vi "podControl_9066.vi"() -> ()   [LabVIEW 2015]
uses:
  <vilib>/platform/TimedLoop/XDataNode/XDataNode.xnode
  <vilib>/Platform/TimedLoop/XDataNode/nitl_modes.ctl
  <vilib>/Platform/TimedLoop/XDataNode/XDNodeRunTimeDep.lvlib
  <vilib>/Platform/TimedLoop/XDataNode/wakeup.ctl
  <vilib>/Platform/TimedLoop/XDataNode/timing_clust.ctl
  podGlobals_9066.vi
  <vilib>/Platform/TimedLoop/XDataNode/loadnilvce.vi
panel:
  out "L:":dbl
  out "Internal Pressure (atm)":dbl(slide) scale=0.0..2.0
  out "Internal Temperature (F)":dbl(slide) scale=50.0..120.0
  out "READY":bool
  out "Runtime (s)":dbl
  in  "START":bool
  out "R:":dbl
  out "Acceleration (m/s^2)":dbl(knob) scale=-30.0..30.0
  out "Position (m)":dbl
  out "Velocity (m/s)":dbl(knob) scale=0.0..300.0
  in  "Custom Profile Velocity (m/s)":dbl
  out "Door Open":bool
  out "Pusher Engaged":bool
  out "Front Brake Engaged":bool
  out "Back Brake Engaged":bool
  in  "Flight Profile":T1(radio)
  out "Progress":u8(slide) caption="Profile Progress" scale=0.0..100.0
  out "Battery Pressure (atm)":dbl(slide) scale=0.0..2.0
  out "Battery Temperature (F)":dbl(slide) scale=50.0..120.0
  in  "STOP":bool
  out "Battery 2 Voltage":dbl(knob) scale=22.0..26.0
  out "Battery 1 Voltage":dbl(knob) scale=22.0..26.0
  # "Z-Height (mm)"
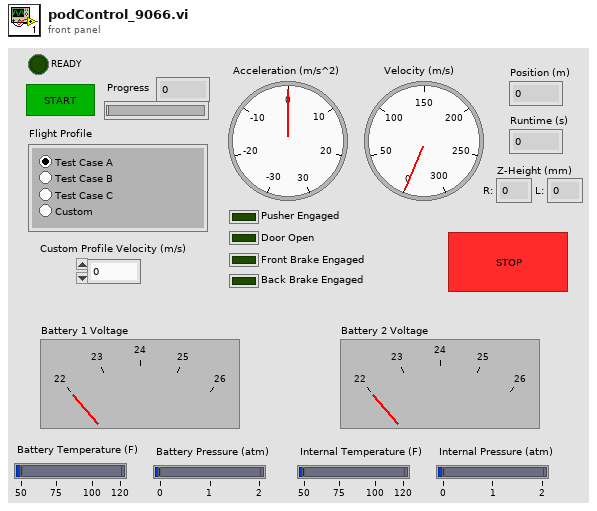
[diagram p1: front panel]
types:
  T1 = enum32{"20 MPH (Test Case A)", "60 MPH (Test Case B)", "150 MPH (Test Case C)", "Custom"}
  T2 = typedef "XDNodeRunTimeDep.lvlib/timing_clust.ctl" = cluster{"Expected End [f-1]":u64, "Actual End [f-1]":u64, "Finished Late? [f-1]":bool, "Expected End [i-1]":u64, "Actual End [i-1]":u64, "Finished Late? [i-1]":bool, "Expected Start [i]":u64, "Actual Start [i]":u64, "Expected Start [f]":u64, "Actual Start [f]":u64, "Source Name":string, "Structure Name":string, "Period":i64, "Deadline":i64, "Offset":i64, "Start":i64, "Priority":i32, "Timeout":i32, "Mode":T3, "Wakeup Reason":T4, "Error":errorcluster, "Source Type":string, "Secondary Source Type":string, "Global End Time":u64, "Global Start Time":u64, "Frame Duration":u64, "Iteration Duration":u64, "Assigned CPU":i32, "I/O Scan Engine Mode":u32}
  T3 = typedef "XDNodeRunTimeDep.lvlib/nitl_modes.ctl" = enum32{"No Change", "Process missed periods, maintain original phase", "Discard missed periods, maintain original phase", "Process missed periods, ignore original phase", "Discard missed periods, ignore original phase"}
  T4 = typedef "XDNodeRunTimeDep.lvlib/wakeup.ctl" = enum32{"Normal", "Aborted", "Asynchronous wakeup", "Timing source error", "Timed loop error", "Timeout"}
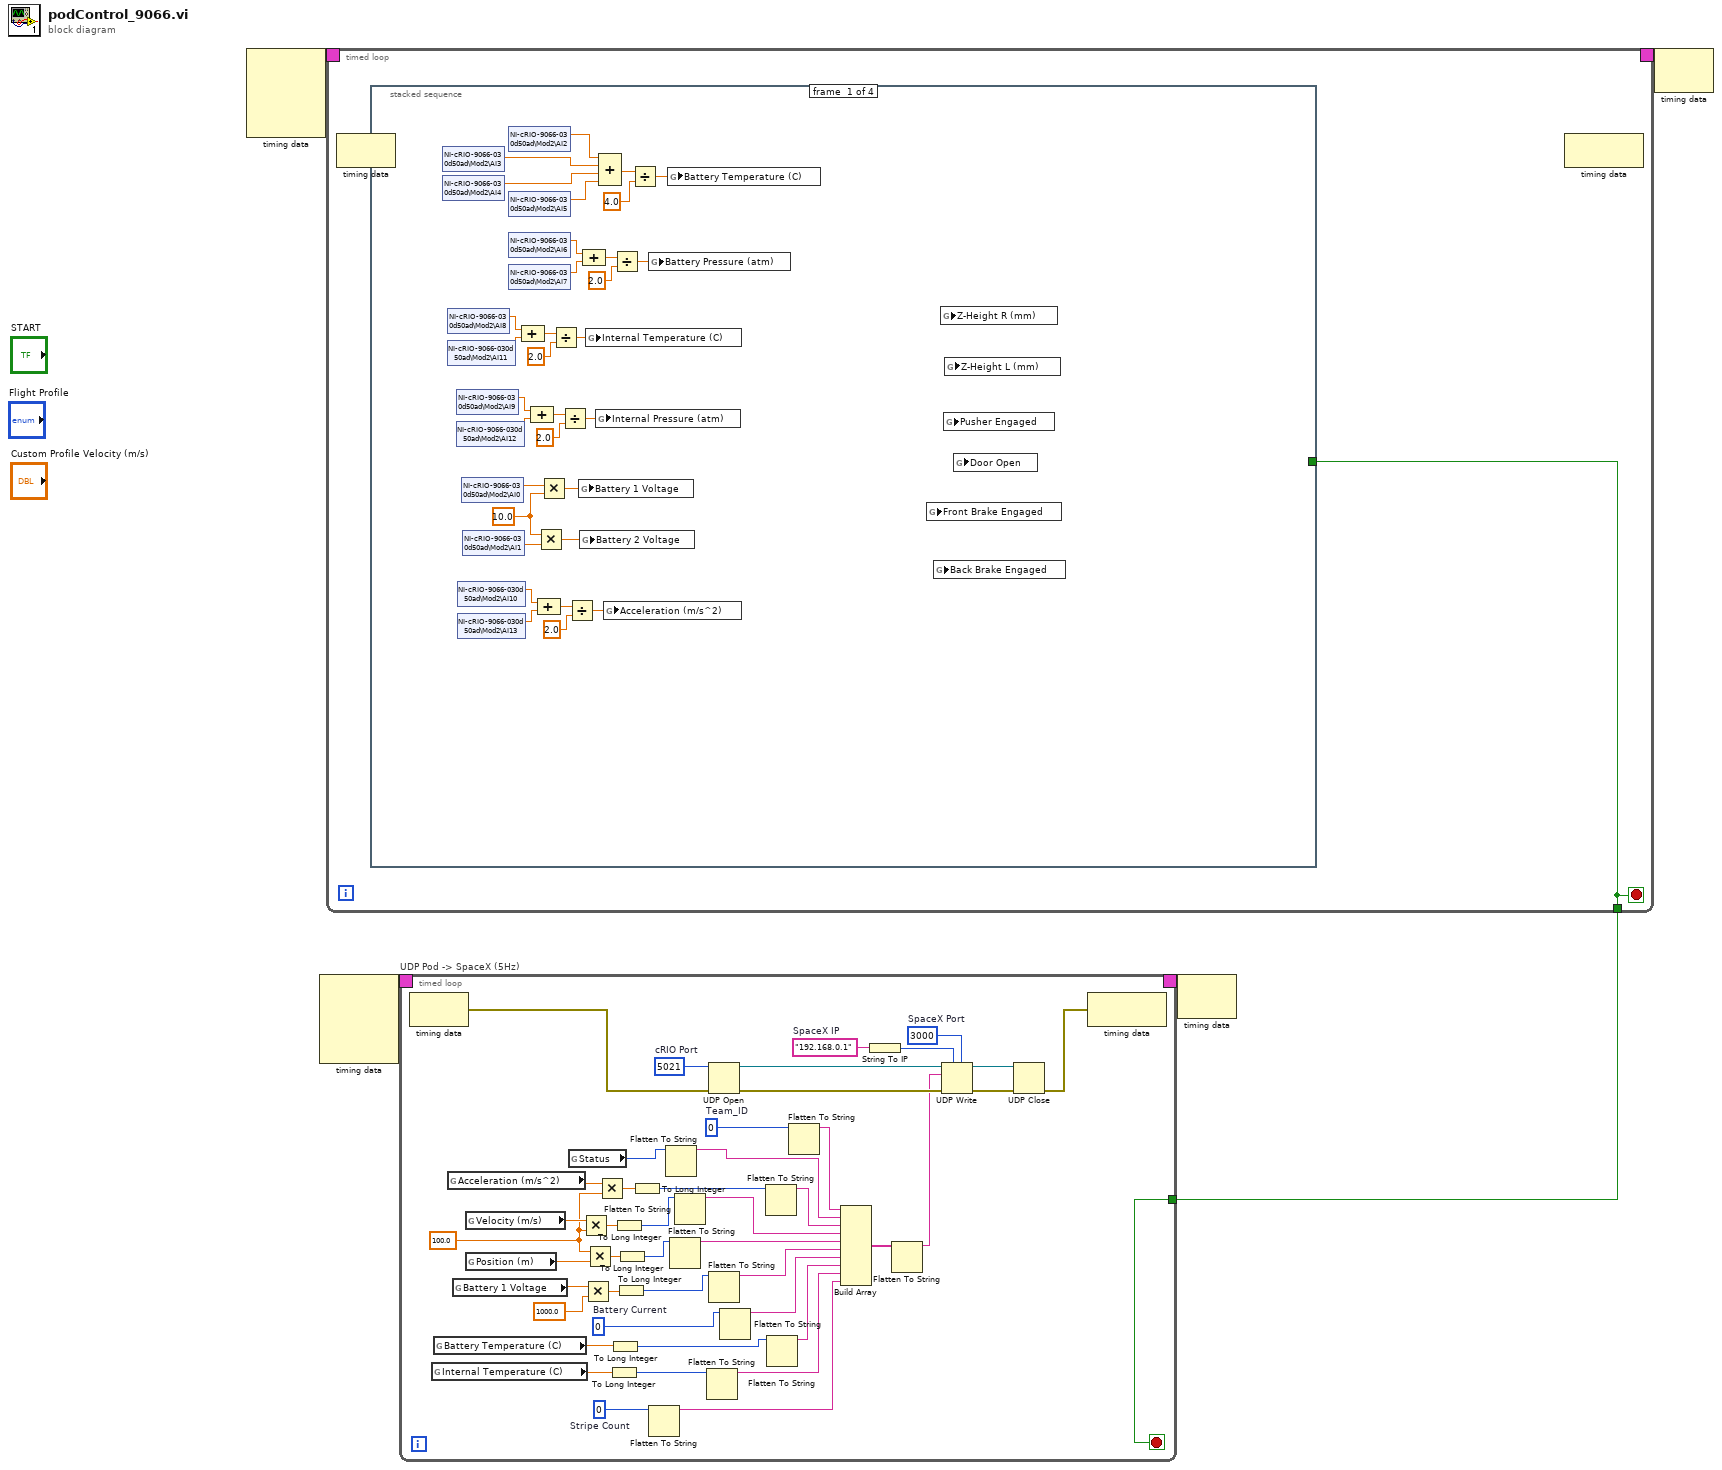
[diagram p0: block diagram]
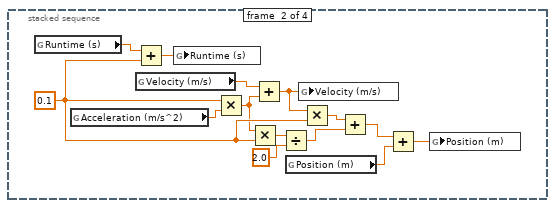
[diagram p2: hidden frame]
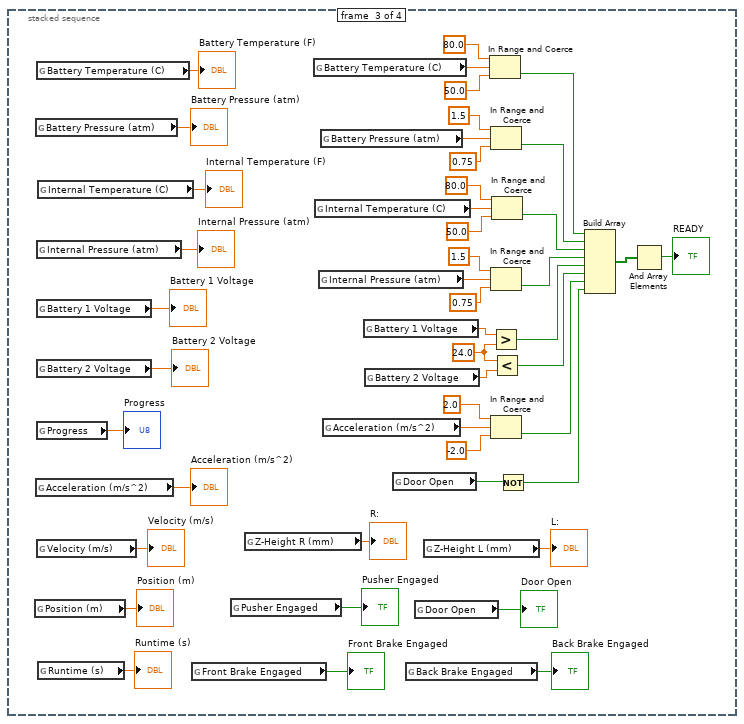
[diagram p3: hidden frame]
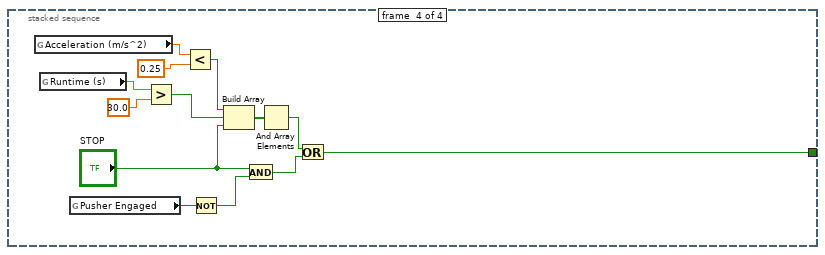
[diagram p4: hidden frame]
diagram:
  n1 = node-c288() -> (w5:T2)  [unwired: 4 in]
  n2 = node-c288() -> (w3:T2)  [unwired: 4 in]
  n3 = timed-loop {
    timing: w5 -> [_]
    timing-out: [_] -> w4
    tunnel: [w6] -> w1
    stop <- w6 stop-if-true
    n4 = node-c288() -> ()  [unwired: 1 in, 1 out]
    n5 = stacked-sequence {
      tunnel: [_ _ _ w106] -> w6
      frame #0 {
        w36 = 10.0
        n6 = shared-variable "NI-cRIO-9066-030d50ad\\Mod2\\AI3"() -> (w19:dbl)  [unwired: 1 in, 1 out]
        n7 = shared-variable "NI-cRIO-9066-030d50ad\\Mod2\\AI4"() -> (w20:dbl)  [unwired: 1 in, 1 out]
        n8 = shared-variable "NI-cRIO-9066-030d50ad\\Mod2\\AI8"() -> (w8:dbl)  [unwired: 1 in, 1 out]
        n9 = shared-variable "NI-cRIO-9066-030d50ad\\Mod2\\AI11"() -> (w9:dbl)  [unwired: 1 in, 1 out]
        n10 = shared-variable "NI-cRIO-9066-030d50ad\\Mod2\\AI9"() -> (w13:dbl)  [unwired: 1 in, 1 out]
        n11 = shared-variable "NI-cRIO-9066-030d50ad\\Mod2\\AI12"() -> (w14:dbl)  [unwired: 1 in, 1 out]
        n12 = shared-variable "NI-cRIO-9066-030d50ad\\Mod2\\AI10"() -> (w29:dbl)  [unwired: 1 in, 1 out]
        n13 = shared-variable "NI-cRIO-9066-030d50ad\\Mod2\\AI13"() -> (w30:dbl)  [unwired: 1 in, 1 out]
        n14 = shared-variable "NI-cRIO-9066-030d50ad\\Mod2\\AI0"() -> (w34:dbl)  [unwired: 1 in, 1 out]
        n15 = shared-variable "NI-cRIO-9066-030d50ad\\Mod2\\AI1"() -> (w35:dbl)  [unwired: 1 in, 1 out]
        n16 = shared-variable "NI-cRIO-9066-030d50ad\\Mod2\\AI2"() -> (w7:dbl)  [unwired: 1 in, 1 out]
        n17 = shared-variable "NI-cRIO-9066-030d50ad\\Mod2\\AI5"() -> (w21:dbl)  [unwired: 1 in, 1 out]
        n18 = shared-variable "NI-cRIO-9066-030d50ad\\Mod2\\AI6"() -> (w24:dbl)  [unwired: 1 in, 1 out]
        n19 = shared-variable "NI-cRIO-9066-030d50ad\\Mod2\\AI7"() -> (w25:dbl)  [unwired: 1 in, 1 out]
        n20 = Compound Arithmetic op=ADD(w8, w9) -> (w10:dbl)
        n21 = Compound Arithmetic op=ADD(w13, w14) -> (w15:dbl)
        n22 = Multiply(x=w36, y=w35) -> (x*y=w38:dbl)
        n23 = Compound Arithmetic op=ADD(w29, w30) -> (w31:dbl)
        n24 = Multiply(x=w34, y=w36) -> (x*y=w37:dbl)
        n25 = Divide(x=w10, y=2.0) -> (x/y=w12:dbl)
        n26 = Divide(x=w15, y=2.0) -> (x/y=w17:dbl)
        n27 = Divide(x=w31, y=2.0) -> (x/y=w33:dbl)
        n28 = global write "podGlobals_9066.vi" "Battery 1 Voltage"(w37) -> ()
        n29 = global write "podGlobals_9066.vi" "Battery 2 Voltage"(w38) -> ()
        n30 = Compound Arithmetic op=ADD(w24, w25) -> (w26:dbl)
        n31 = global write "podGlobals_9066.vi" "Internal Temperature (C)"(w12) -> ()
        n32 = global write "podGlobals_9066.vi" "Internal Pressure (atm)"(w17) -> ()
        n33 = Compound Arithmetic op=ADD(w7, w19, w20, w21) -> (w18:dbl)
        n34 = global write "podGlobals_9066.vi" "Acceleration (m/s^2)"(w33) -> ()
        n35 = Divide(x=w26, y=2.0) -> (x/y=w28:dbl)
        n36 = Divide(x=w18, y=4.0) -> (x/y=w23:dbl)
        n37 = global write "podGlobals_9066.vi" "Battery Pressure (atm)"(w28) -> ()
        n38 = global write "podGlobals_9066.vi" "Battery Temperature (C)"(w23) -> ()
        n39 = global read "podGlobals_9066.vi" "Front Brake Engaged"() -> ()  [unwired: 1 in]
        n40 = global read "podGlobals_9066.vi" "Back Brake Engaged"() -> ()  [unwired: 1 in]
        n41 = global read "podGlobals_9066.vi" "Z-Height R (mm)"() -> ()  [unwired: 1 in]
        n42 = global read "podGlobals_9066.vi" "Pusher Engaged"() -> ()  [unwired: 1 in]
        n43 = global read "podGlobals_9066.vi" "Z-Height L (mm)"() -> ()  [unwired: 1 in]
        n44 = global read "podGlobals_9066.vi" "Door Open"() -> ()  [unwired: 1 in]
      }
      frame #1 {
        w51 = 0.1
        n45 = global read "podGlobals_9066.vi" "Runtime (s)"() -> (w40:dbl)
        n46 = global read "podGlobals_9066.vi" "Acceleration (m/s^2)"() -> (w49:dbl)
        n47 = Add(x=w40, y=w51) -> (x+y=w39:dbl)
        n48 = global read "podGlobals_9066.vi" "Velocity (m/s)"() -> (w41:dbl)
        n49 = global write "podGlobals_9066.vi" "Runtime (s)"(w39) -> ()
        n50 = Multiply(x=w51, y=w49) -> (x*y=w43:dbl)
        n51 = Multiply(x=w43, y=w51) -> (x*y=w44:dbl)
        n52 = Add(x=w41, y=w43) -> (x+y=w52:dbl)
        n53 = Divide(x=w44, y=2.0) -> (x/y=w47:dbl)
        n54 = global read "podGlobals_9066.vi" "Position (m)"() -> (w46:dbl)
        n55 = global write "podGlobals_9066.vi" "Velocity (m/s)"(w52) -> ()
        n56 = Multiply(x=w52, y=w51) -> (x*y=w50:dbl)
        n57 = Add(x=w50, y=w47) -> (x+y=w48:dbl)
        n58 = Add(x=w48, y=w46) -> (x+y=w42:dbl)
        n59 = global write "podGlobals_9066.vi" "Position (m)"(w42) -> ()
      }
      frame #2 {
        w72 = 24.0
        n60 = global read "podGlobals_9066.vi" "Position (m)"() -> (→"Position (m)":dbl)
        n61 = global read "podGlobals_9066.vi" "Battery Pressure (atm)"() -> (→"Battery Pressure (atm)":dbl)
        n62 = global read "podGlobals_9066.vi" "Acceleration (m/s^2)"() -> (→"Acceleration (m/s^2)":dbl)
        n63 = global read "podGlobals_9066.vi" "Battery Temperature (C)"() -> (→"Battery Temperature (F)":dbl)
        n64 = global read "podGlobals_9066.vi" "Internal Pressure (atm)"() -> (→"Internal Pressure (atm)":dbl)
        n65 = global read "podGlobals_9066.vi" "Battery 1 Voltage"() -> (→"Battery 1 Voltage":dbl)
        n66 = global read "podGlobals_9066.vi" "Battery 2 Voltage"() -> (→"Battery 2 Voltage":dbl)
        n67 = global read "podGlobals_9066.vi" "Progress"() -> (→"Progress":dbl)
        n68 = global read "podGlobals_9066.vi" "Velocity (m/s)"() -> (→"Velocity (m/s)":dbl)
        n69 = global read "podGlobals_9066.vi" "Internal Temperature (C)"() -> (→"Internal Temperature (F)":dbl)
        n70 = global read "podGlobals_9066.vi" "Runtime (s)"() -> (→"Runtime (s)":dbl)
        n71 = global read "podGlobals_9066.vi" "Front Brake Engaged"() -> (→"Front Brake Engaged":bool)
        n72 = global read "podGlobals_9066.vi" "Pusher Engaged"() -> (→"Pusher Engaged":bool)
        n73 = global read "podGlobals_9066.vi" "Z-Height R (mm)"() -> (→"R:":dbl)
        n74 = global read "podGlobals_9066.vi" "Battery Temperature (C)"() -> (w61:dbl)
        n75 = global read "podGlobals_9066.vi" "Internal Temperature (C)"() -> (w55:dbl)
        n76 = global read "podGlobals_9066.vi" "Internal Pressure (atm)"() -> (w58:dbl)
        n77 = global read "podGlobals_9066.vi" "Battery Pressure (atm)"() -> (w64:dbl)
        n78 = global read "podGlobals_9066.vi" "Acceleration (m/s^2)"() -> (w67:dbl)
        n79 = global read "podGlobals_9066.vi" "Battery 1 Voltage"() -> (w70:dbl)
        n80 = global read "podGlobals_9066.vi" "Battery 2 Voltage"() -> (w71:dbl)
        n81 = global read "podGlobals_9066.vi" "Door Open"() -> (w80:bool)
        n82 = global read "podGlobals_9066.vi" "Back Brake Engaged"() -> (→"Back Brake Engaged":bool)
        n83 = global read "podGlobals_9066.vi" "Door Open"() -> (→"Door Open":bool)
        n84 = global read "podGlobals_9066.vi" "Z-Height L (mm)"() -> (→"L:":dbl)
        n85 = In Range and Coerce(upper limit=80.0, x=w61, lower limit=50.0) -> (In Range?=w73:bool)  [unwired: 1 out]
        n86 = In Range and Coerce(upper limit=1.5, x=w64, lower limit=0.75) -> (In Range?=w74:bool)  [unwired: 1 out]
        n87 = In Range and Coerce(upper limit=1.5, x=w58, lower limit=0.75) -> (In Range?=w76:bool)  [unwired: 1 out]
        n88 = Greater?(x=w70, y=w72) -> (0:w77:bool)
        n89 = In Range and Coerce(upper limit=2.0, x=w67, lower limit=-2.0) -> (In Range?=w79:bool)  [unwired: 1 out]
        n90 = In Range and Coerce(upper limit=80.0, x=w55, lower limit=50.0) -> (In Range?=w75:bool)  [unwired: 1 out]
        n91 = Less?(x=w72, y=w71) -> (x < y?=w78:bool)
        n92 = Not(x=w80) -> (.not. x?=w81:bool)
        n93 = Build Array(w73, w74, w75, w76, w77, w78, w79, w81) -> (w53:bool[])
        n94 = And Array Elements(Boolean array=w53) -> (logical AND=→"READY":bool)
      }
      frame #3 {
        n95 = global read "podGlobals_9066.vi" "Acceleration (m/s^2)"() -> (w103:dbl)
        n96 = global read "podGlobals_9066.vi" "Runtime (s)"() -> (w108:dbl)
        n97 = global read "podGlobals_9066.vi" "Pusher Engaged"() -> (w111:bool)
        n98 = Greater?(x=w108, y=30.0) -> (0:w101:bool)
        n99 = Less?(x=w103, y=0.25) -> (x < y?=w99:bool)
        n100 = Not(x=w111) -> (.not. x?=w110:bool)
        n101 = Build Array(w99, w101, "STOP") -> (w105:bool[])
        n102 = And(x="STOP", y=w110) -> (x .and. y?=w109:bool)
        n103 = And Array Elements(Boolean array=w105) -> (logical AND=w104:bool)
        n104 = Or(x=w104, y=w109) -> (x .or. y?=w106:bool)
      }
    }
    n105 = node-c288() -> ()  [unwired: 1 in, 1 out]
  }
  n106 = timed-loop "UDP Pod -> SpaceX (5Hz)" {
    timing: w3 -> [_]
    timing-out: [_] -> w2
    tunnel: w1 -> [w114]
    stop <- w114 stop-if-true
    w119 = u32 0  # Stripe Count
    w125 = 0  # Battery Current
    w146 = 100.0
    w137 = u8 0  # Team_ID
    w151 = 3000  # SpaceX Port
    w115 = "192.168.0.1"  # SpaceX IP
    w154 = 5021  # cRIO Port
    n107 = node-c288() -> (w158:errorcluster)  [unwired: 1 in]
    n108 = global read "podGlobals_9066.vi" "Internal Temperature (C)"() -> (w138:dbl)
    n109 = global read "podGlobals_9066.vi" "Battery Temperature (C)"() -> (w139:dbl)
    n110 = global read "podGlobals_9066.vi" "Acceleration (m/s^2)"() -> (w149:dbl)
    n111 = global read "podGlobals_9066.vi" "Battery 1 Voltage"() -> (w140:dbl)
    n112 = global read "podGlobals_9066.vi" "Velocity (m/s)"() -> (w148:dbl)
    n113 = global read "podGlobals_9066.vi" "Position (m)"() -> (w147:dbl)
    n114 = global read "podGlobals_9066.vi" "Status"() -> (w135:u8)
    n115 = Multiply(x=w148, y=w146) -> (x*y=w144:dbl)
    n116 = Multiply(x=w140, y=1000.0) -> (x*y=w142:dbl)
    n117 = Multiply(x=w146, y=w147) -> (x*y=w143:dbl)
    n118 = Multiply(x=w149, y=w146) -> (x*y=w145:dbl)
    n119 = To Long Integer(number=w138) -> (32bit integer=w121:i32)
    n120 = To Long Integer(number=w139) -> (32bit integer=w123:i32)
    n121 = To Long Integer(number=w144) -> (32bit integer=w130:i32)
    n122 = To Long Integer(number=w142) -> (32bit integer=w127:i32)
    n123 = To Long Integer(number=w143) -> (32bit integer=w128:i32)
    n124 = To Long Integer(number=w145) -> (32bit integer=w132:i32)
    n125 = Flatten To String(anything=w119) -> (data string=w118:string)  [unwired: 3 in, 2 out]
    n126 = Flatten To String(anything=w135) -> (data string=w134:string)  [unwired: 3 in, 2 out]
    n127 = Flatten To String(anything=w128) -> (data string=w129:string)  [unwired: 3 in, 2 out]
    n128 = Flatten To String(anything=w130) -> (data string=w131:string)  [unwired: 3 in, 2 out]
    n129 = Flatten To String(anything=w121) -> (data string=w120:string)  [unwired: 3 in, 2 out]
    n130 = UDP Open(8:w158, 11:w154) -> (port=w153:refnum<k16>, 0:w157:errorcluster)  [unwired: 3 in, 1 out]
    n131 = Flatten To String(anything=w127) -> (data string=w126:string)  [unwired: 3 in, 2 out]
    n132 = Flatten To String(anything=w125) -> (data string=w124:string)  [unwired: 3 in, 2 out]
    n133 = Flatten To String(anything=w132) -> (data string=w133:string)  [unwired: 3 in, 2 out]
    n134 = Flatten To String(anything=w123) -> (data string=w122:string)  [unwired: 3 in, 2 out]
    n135 = Flatten To String(anything=w137) -> (data string=w136:string)  [unwired: 3 in, 2 out]
    n136 = Build Array(w136, w134, w133, w131, w129, w126, w124, w122, w120, w118) -> (w117:string[])
    n137 = String To IP(1:w115) -> (0:w152:u32)
    n138 = Flatten To String(anything=w117) -> (data string=w116:string)  [unwired: 3 in, 2 out]
    n139 = UDP Write(address=w152, port or service name=w151, connection ID=w153, data in=w116, 8:w157) -> (error out=w156:errorcluster, 3:w150:refnum<k16>)  [unwired: 1 in]
    n140 = UDP Close(connection ID=w150, 8:w156) -> (error out=w155:errorcluster)  [unwired: 1 out]
    n141 = node-c288(w155) -> ()  [unwired: 1 out]
  }
  n142 = node-c288(w2) -> ()  [unwired: 1 out]
  n143 = node-c288(w4) -> ()  [unwired: 1 out]
